vi "TESTE_PRESSAO_OFICINA.vi"() -> (0 "Pressão 2":dbl format="%0.2f", 3 "Pressão 1":dbl format="%0.2f")   [LabVIEW 2019]
uses:
  <vilib>/DAQmx/read.llb/DAQmx Read (Analog 2D DBL NChan NSamp).vi
  <vilib>/Analysis/baseanly.llb/Mean (DBL).vi
  <vilib>/DAQmx/configure/timing.llb/DAQmx Timing (Sample Clock).vi
  <vilib>/DAQmx/miscellaneous.llb/DAQmx Fill In Error Info.vi
  <vilib>/Analysis/NI_AALBase.lvlib
panel:
  out "DAQmx Task Name":refnum<k21>="Teste_oficina_Tensao"
  in  "Numero de pontos adquiridos por segundo":dbl=1000.0 format="%0.2f"
  out "Waveform Graph":dbl[][](graph)
  out "error out":errorcluster
  # "VI destinada a testes anteriores na oficina\nVI etsá absoleta. nao utilizar ela"
  # "/s"
  # "mmH2O"
  # "mmH2O"
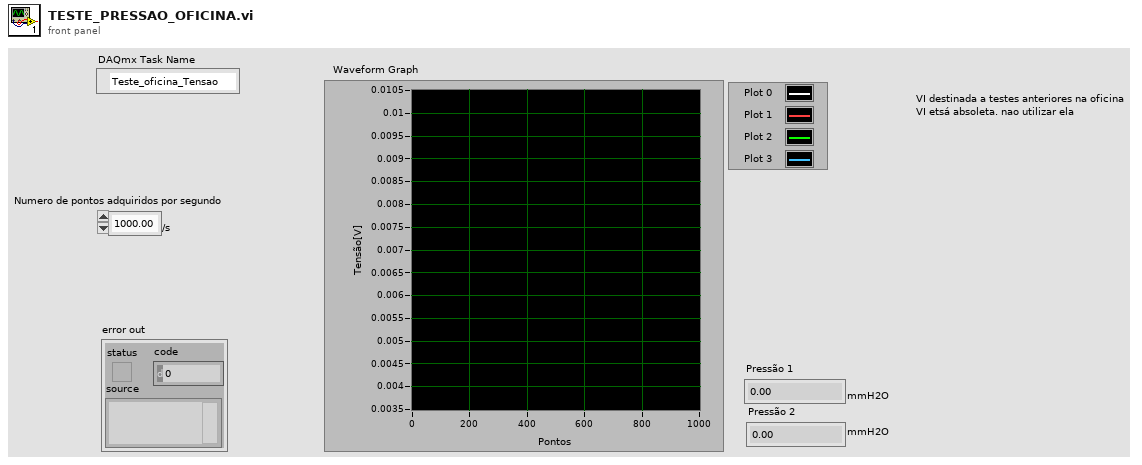
[diagram p1: front panel]
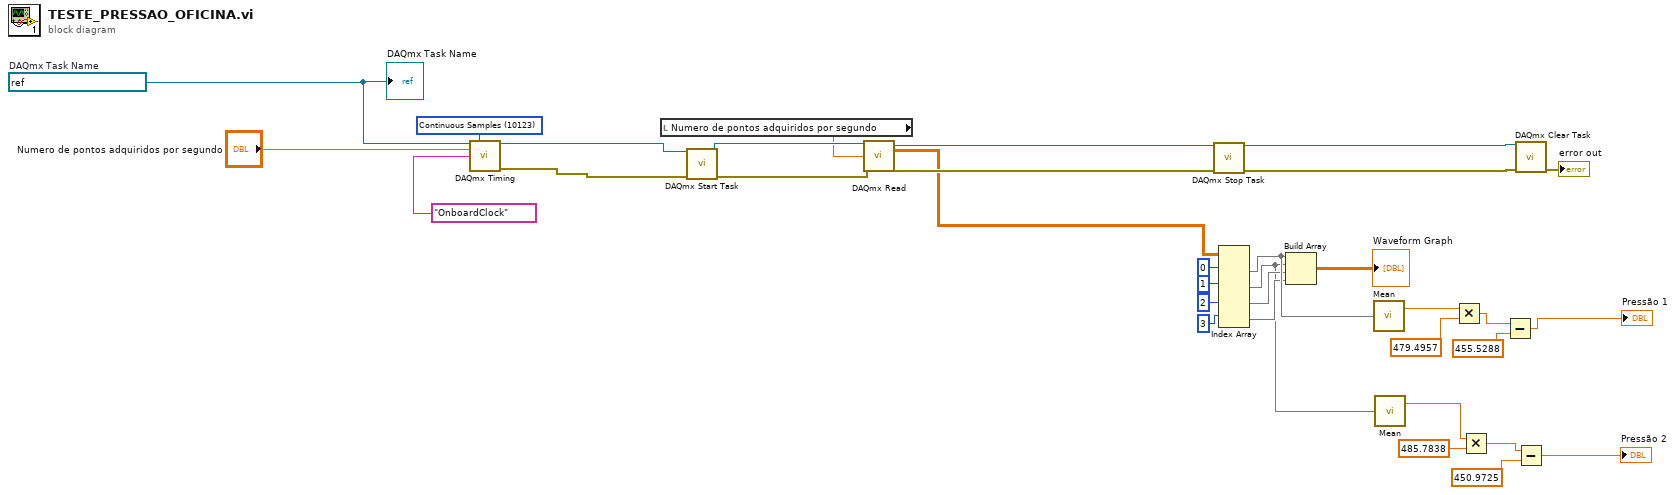
[diagram p0: block diagram]
diagram:
  w27 = refnum<k21> "Teste_oficina_Tensao"  # DAQmx Task Name
  w34 = 10123 items=["Finite Samples"=10178, "Continuous Samples"=10123, "Hardware Timed Single Point"=12522] ("sample mode")
  n1 = call-poly <vilib>:"DAQmx Timing.vi"("task/channels in"=w27, "sample mode"=w34, "rate"="Numero de pontos adquiridos por segundo", "source"=tag "OnboardClock") -> ("task out"=w33:refnum<k21>, "error out"=w32:errorcluster)  [unwired: 10 in]
  n2 = local read "Numero de pontos adquiridos por segundo"() -> (w12:dbl)
  n3 = call <vilib>:"DAQmx Start Task.vi"("task/channels in"=w33, "error in"=w32) -> ("task out"=w26:refnum<k21>, "error out"=w25:errorcluster)  [unwired: 12 in]
  n4 = call-poly <vilib>:"DAQmx Read.vi"("task/channels in"=w26, "number of samples per channel"=w12, "error in"=w25) -> ("task out"=w24:refnum<k21>, "data"=w14:dbl[][], "error out"=w23:errorcluster)  [unwired: 10 in]
  n5 = call <vilib>:"DAQmx Stop Task.vi"("task/channels in"=w24, "error in"=w23) -> ("task out"=w30:refnum<k21>, "error out"=w31:errorcluster)  [unwired: 12 in]
  n6 = Index Array(array=w14, index (row) #1=0 ("index (row)"), index (row) #2=1 ("index (row)"), index (row) #3=2 ("index (row)"), index (row) #4=3 ("disabled index (col)")) -> (element #1=w17:dbl[], element #2=w5:dbl[], element #3=w16:dbl[], element #4=w15:dbl[])  [unwired: 4 in]
  n7 = Build Array(w17, w5, w16, w15) -> (→"Waveform Graph":dbl[][])
  n8 = call-poly <vilib>:"Mean.vi"("X"=w17) -> ("mean"=w4:dbl)  [unwired: 1 out]
  n9 = call-poly <vilib>:"Mean.vi"("X"=w5) -> ("mean"=w3:dbl)  [unwired: 1 out]
  n10 = Multiply(x=w4, y=479.4957) -> (x*y=w9:dbl)
  n11 = Multiply(x=w3, y=485.7838) -> (x*y=w7:dbl)
  n12 = Subtract(x=w9, y=455.5288) -> (x-y=→"Pressão 1":dbl)
  n13 = call <vilib>:"DAQmx Clear Task.vi"("task in"=w30, "error in"=w31) -> ("error out"=→"error out":errorcluster)  [unwired: 13 in]
  n14 = Subtract(x=w7, y=450.9725) -> (x-y=→"Pressão 2":dbl)
  "DAQmx Task Name" <- w27
